vi "Read_and_plot_files.vi"() -> ()   [LabVIEW 2016]
uses:
  <vilib>/Utility/miscctls.llb/LVStringsAndValuesArrayTypeDef_U16.ctl
panel:
  in  "Enum":enum16{"fffsa", "ff", "3", "ds", "sds"}(ring)
  out "Strings []":string[](array[string])
  out "Number of Items":u32
  out "Enum 3":enum16{"fffsa", "ff", "3", "ds", "sds"}(ring)
  in  "Ring":u16(ring) items=["3123"=1, "Eple"=2, "dasda"=3, "sada"=4]
  out "Ring 2":u16(ring)
  in  "Strings And Values []":T1
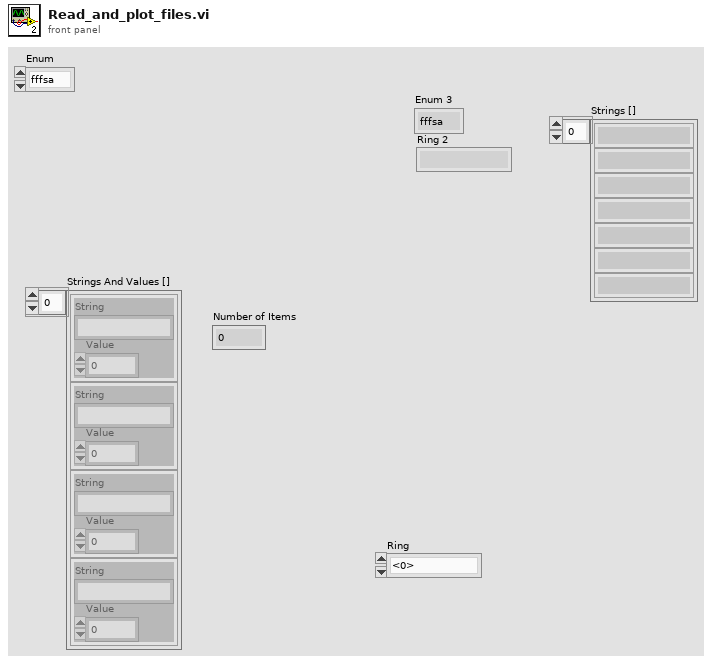
[diagram p1: front panel]
types:
  T1 = typedef "LVStringsAndValuesArrayTypeDef_U16.ctl" = cluster{"String":string, "Value":u16}[]
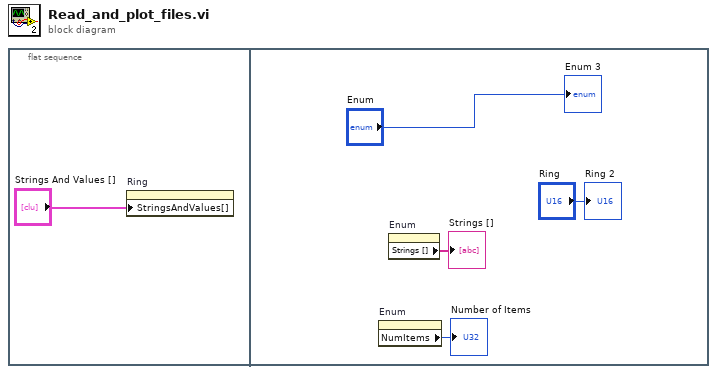
[diagram p0: block diagram]
diagram:
  n1 = flat-sequence {
    frame #0 {
      n2 = property on="Ring" class="Ring (strict)"("StringsAndValues[]"="Strings And Values []") -> ()  [unwired: 2 in, 2 out]
    }
    frame #1 {
      n3 = property on="Enum" class="Enum (strict)"() -> ("NumItems"=→"Number of Items":u32)  [unwired: 2 in, 2 out]
      n4 = property on="Enum" class="Enum (strict)"() -> ("Strings []"=→"Strings []":string[])  [unwired: 2 in, 2 out]
      "Enum 3" <- "Enum"
      "Ring 2" <- "Ring"
    }
  }
